vi "SetPath.vi"(8 "ErrorIn":errorcluster caption="Error In(no Error)", 10 "Path":path caption="Attribute1", 11 "ReferenceIn":refnum<class "ErrorDefinitionSQLite.lvclass"> caption="Reference In") -> (0 "ErrorOut":errorcluster caption="Error Out", 3 "ReferenceOut":refnum<class "ErrorDefinitionSQLite.lvclass"> caption="Reference Out")   [LabVIEW 2018, in "ErrorDefinitionSQLite.lvclass"]
uses:
  <userlib>/_express/CustomErrorCreator/ErrorDefinitionSQLite/ErrorDefinitionSQLite.lvclass
  <vilib>/drjdpowell/SQLite Library/SQL Connection/Open (path).vi
  <vilib>/drjdpowell/SQLite Library/SQL Connection/Open (string).vi
  <vilib>/AdvancedString/Path To Command Line String.vi
  <vilib>/drjdpowell/SQLite Library/SQL Connection/Execute SQL (No results).vi
  <vilib>/drjdpowell/SQLite Library/SQL Connection/Connection.lvclass
  <vilib>/drjdpowell/SQLite Library/SQLite.lvlib
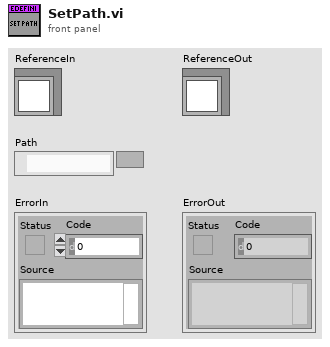
[diagram p1: front panel]
types:
  T1 = enum16{"New or existing", "Existing", "Read only"}
  T2 = typedef "ErrorDefinitionSQLite.lvclass/ObjectAttributes.ctl" = cluster{"Path":path}
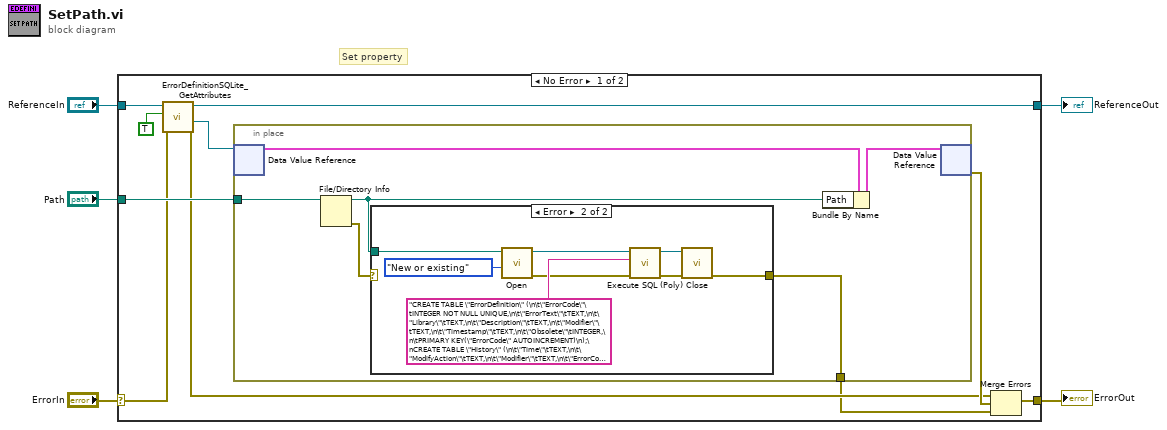
[diagram p0: block diagram]
diagram:
  # "Set property"
  n1 = case shown="No Error" "ErrorIn" {
    selector: "ErrorIn" -> [w9 w32]
    tunnel: [w13 w32] -> w4
    tunnel: [w11 w31] -> w2
    tunnel: "ReferenceIn" -> [w12 w31]
    tunnel: "Path" -> [w15 _]
    frame No Error {
      n2 = call <userlib>:"ErrorDefinitionSQLite_GetAttributes.vi"("ErrorIn"=w9, "OnlyGetDVRReference"=TRUE ("OnlyGetDvrReference(False)"), "Reference in"=w12) -> ("ErrorOut"=w8:errorcluster, "DataRef"=w10:refnum<data-value>, "Reference out"=w11:refnum<class "ErrorDefinitionSQLite.lvclass">)  [unwired: 5 in, 1 out]
      n3 = in-place {
        in-place-border: w15 -> [w19]
        in-place-border: [w16] -> w6
        n4 = in-place-dvr #1(w10) -> (w21:T2)  [unwired: 1 out]
        n5 = File/Directory Info(path=w19) -> (path out=w17:path, error out=w18:errorcluster)  [unwired: 1 in, 5 out]
        n6 = case shown="Error" w18 {
          selector: w18 -> [w22 _]
          tunnel: w17 -> [_ w30]
          tunnel: [w22 w23] -> w16
          frame No Error {
          }
          frame Error {
            n7 = call-poly <vilib>:"Open.vi"("File Option"=T1."New or existing", "db file"=w30) -> ("error out"=w24:errorcluster, "SQLite Connection"=w28:refnum<class "Connection.lvclass">)  [unwired: 8 in]
            n8 = call-poly <vilib>:"Execute SQL (Poly).vi"("error in (no error)"=w24, "SQL"="CREATE TABLE \"ErrorDefinition\" (\n\t\"ErrorCode\"\tINTEGER NOT NULL UNIQUE,\n\t\"ErrorText\"\tTEXT,\n\t\"Library\"\tTEXT,\n\t\"Description\"\tTEXT,\n\t\"Modifier\"\tTEXT,\n\t\"Timestamp\"\tTEXT,\n\t\"Obsolete\"\tINTEGER,\n\tPRIMARY KEY(\"ErrorCode\" AUTOINCREMENT)\n);\nCREATE TABLE \"History\" (\n\t\"Time\"\tTEXT,\n\t\"ModifyAction\"\tTEXT,\n\t\"Modifier\"\tTEXT,\n\t\"ErrorCode\"\tINTEGER,\n\t\"ErrorText\"\tTEXT,\n\t\"Library\"\tTEXT,\n\t\"Description\"\tTEXT\n);\nINSERT INTO ErrorDefinition (ErrorCode, ErrorText)\nVALUES ( 500000, \"Generic Error\") ", "SQLite Connection in"=w28) -> ("error out"=w26:errorcluster, "SQLite Connection"=w25:refnum<class "Connection.lvclass">)  [unwired: 7 in]
            n9 = call-dynamic "Close.vi"("error in (no error)"=w26, "SQLite Connection in"=w25) -> ("error out"=w23:errorcluster)  [unwired: 9 in]
          }
        }
        n10 = Bundle By Name(cluster=w21, "Path"=w17) -> (w20:T2)
        n11 = in-place-dvr #1(w20) -> (w14:errorcluster)  [unwired: 1 out]
      }
      n12 = Merge Errors(w8, w14, w6) -> (w13:errorcluster)
    }
    frame Error {
    }
  }
  "ErrorOut" <- w4
  "ReferenceOut" <- w2
